vi "Configure Timed Output.vi"(7 "Channel (1:1)":u16(ring)=1 items=["1"=1, "2"=2, "3"=3], 8 "error in (no error)":errorcluster, 9 "Time (1s)":dbl=1.0 min=0.0 max=99999.9 step=1.0 format="%.1f", 10 "Enable Timer Output (F: False)":bool, 11 "VISA resource name":refnum<visa-resource-name>) -> (0 "error out":errorcluster, 3 "VISA resource name out":refnum<visa-resource-name>)   [LabVIEW 2017, in "BK Precision 913XX.lvlib"]
doc: "Configures and enables the internal output timer of the selected channel."
uses:
  <instrlib>/BK Precision 913XX/BK Precision 913XX.lvlib
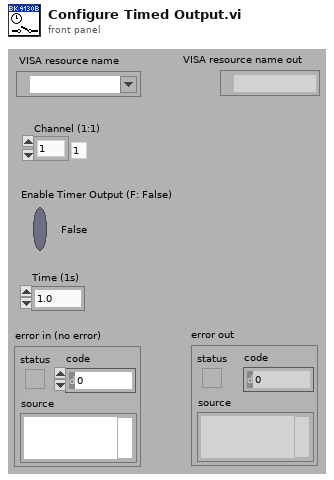
[diagram p1: front panel]
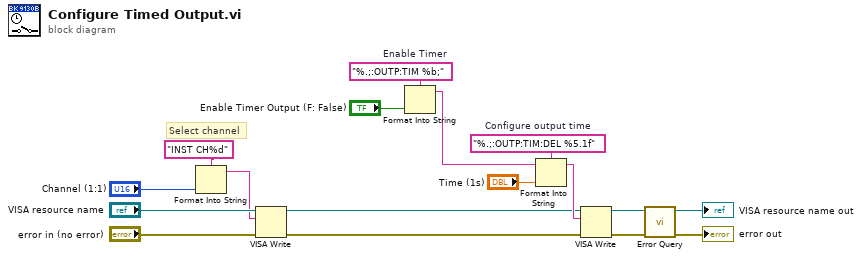
[diagram p0: block diagram]
diagram:
  w12 = "%.;:OUTP:TIM:DEL %5.1f"  # Configure output time
  w15 = "%.;:OUTP:TIM %b;"  # Enable Timer
  # "Select channel"
  n1 = Format Into String(format string="INST CH%d", "Channel (1:1)") -> (resulting string=w2:string)  [unwired: 2 in, 1 out]
  n2 = VISA Write(VISA resource name="VISA resource name", write buffer=w2, error in (no error)="error in (no error)") -> (VISA resource name out=w4:refnum<visa-resource-name>, error out=w5:errorcluster)  [unwired: 1 out]
  n3 = Format Into String(format string=w15, "Enable Timer Output (F: False)") -> (resulting string=w10:string)  [unwired: 2 in, 1 out]
  n4 = Format Into String(format string=w12, initial string=w10, "Time (1s)") -> (resulting string=w9:string)  [unwired: 1 in, 1 out]
  n5 = VISA Write(VISA resource name=w4, write buffer=w9, error in (no error)=w5) -> (VISA resource name out=w14:refnum<visa-resource-name>, error out=w13:errorcluster)  [unwired: 1 out]
  n6 = call <instrlib>:"Error Query.vi"("error in (no error)"=w13, "VISA resource name"=w14) -> ("error out"=→"error out":errorcluster, "VISA resource name out"=→"VISA resource name out":refnum<visa-resource-name>)  [unwired: 6 in, 2 out]
